vi "AutoCAD NET cmds.vi"(6 "AutoCAD cmd":T3, 8 "error in (no error)":errorcluster, 9 "progress":refnum<vi>, 10 "Mathcad Output":T2, 11 "DesignRequest":T1) -> (0 "error out":errorcluster, 3 "DesignRequest out":T1)   [LabVIEW 2012, in "Design Server.lvlib"]
uses:
  Design Server.lvlib
  AutoCAD cmds.ctl
  Design Request.ctl
  Variable cluster.ctl
  C:/Program Files/Autodesk/AutoCAD 2013/Autodesk.AutoCAD.Interop.dll
  Program Files/Autodesk/AutoCAD 2013/Autodesk.AutoCAD.Interop.dll
panel:
  out "error out 3":errorcluster
  out "error out 2":errorcluster
  out "error array":errorcluster[](array[cluster])
  out "Version":string
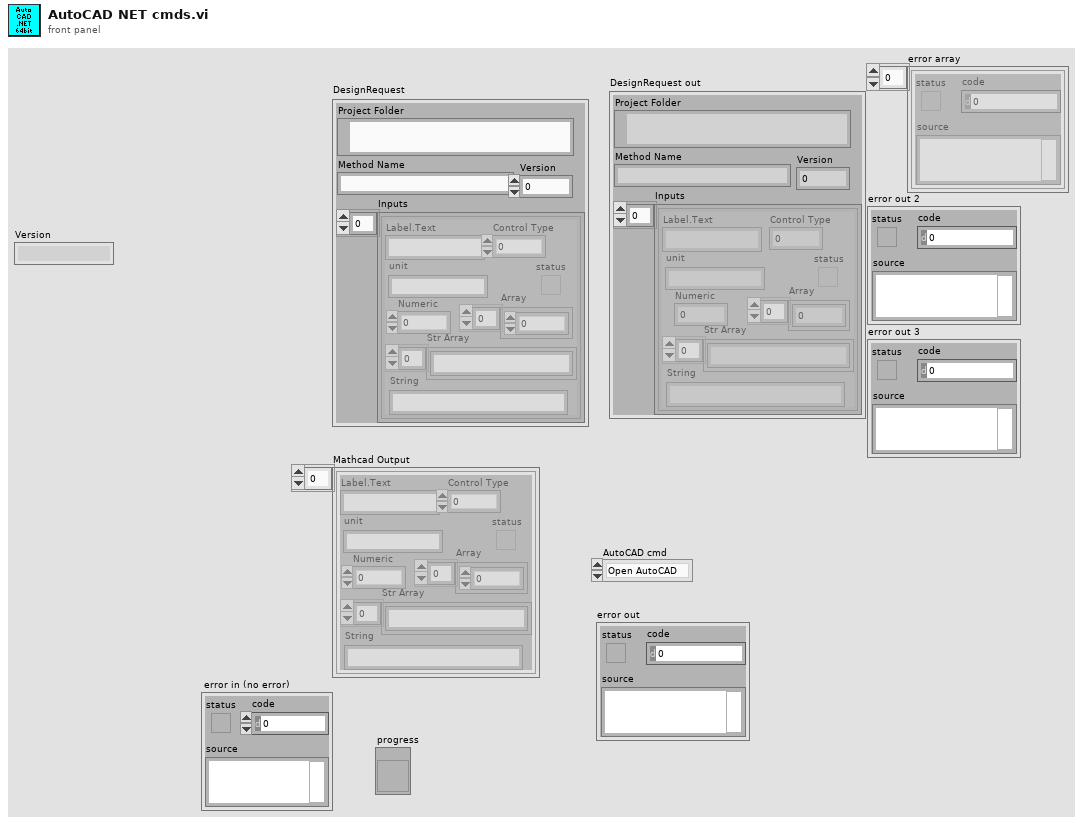
[diagram p1: front panel]
types:
  T1 = typedef "Design Server.lvlib/Design Request.ctl" = cluster{"Project Folder":path, "Method Name":string, "Inputs":T2, "Version":i32}
  T2 = typedef "Design Server.lvlib/Variable cluster.ctl" = cluster{"Label.Text":string, "Control Type":u32, "Numeric":dbl, "Array":dbl[], "status":bool, "Str Array":string[], "String":string, "unit":string}[]
  T3 = typedef "Design Server.lvlib/AutoCAD cmds.ctl" = enum16{"Open AutoCAD", "Create Drawing", "Quit"}
  T4 = typedef "Method.ctl" = cluster{"Title":string, "About":string, "Input Parameters":cluster{"Description":string, "Name":string, "Min":string, "Max":string, "Default":string, "Units":string, "Increment":string, "Stock designs":string[]}[], "AutoCAD drawings":cluster{"File Name":string, "AC Variables":string[]}[], "Stock file names":string[], "Publish files":string[], "Display images":string[]}
  T5 = cluster{"File Name":string, "AC Variables":string[]}[]
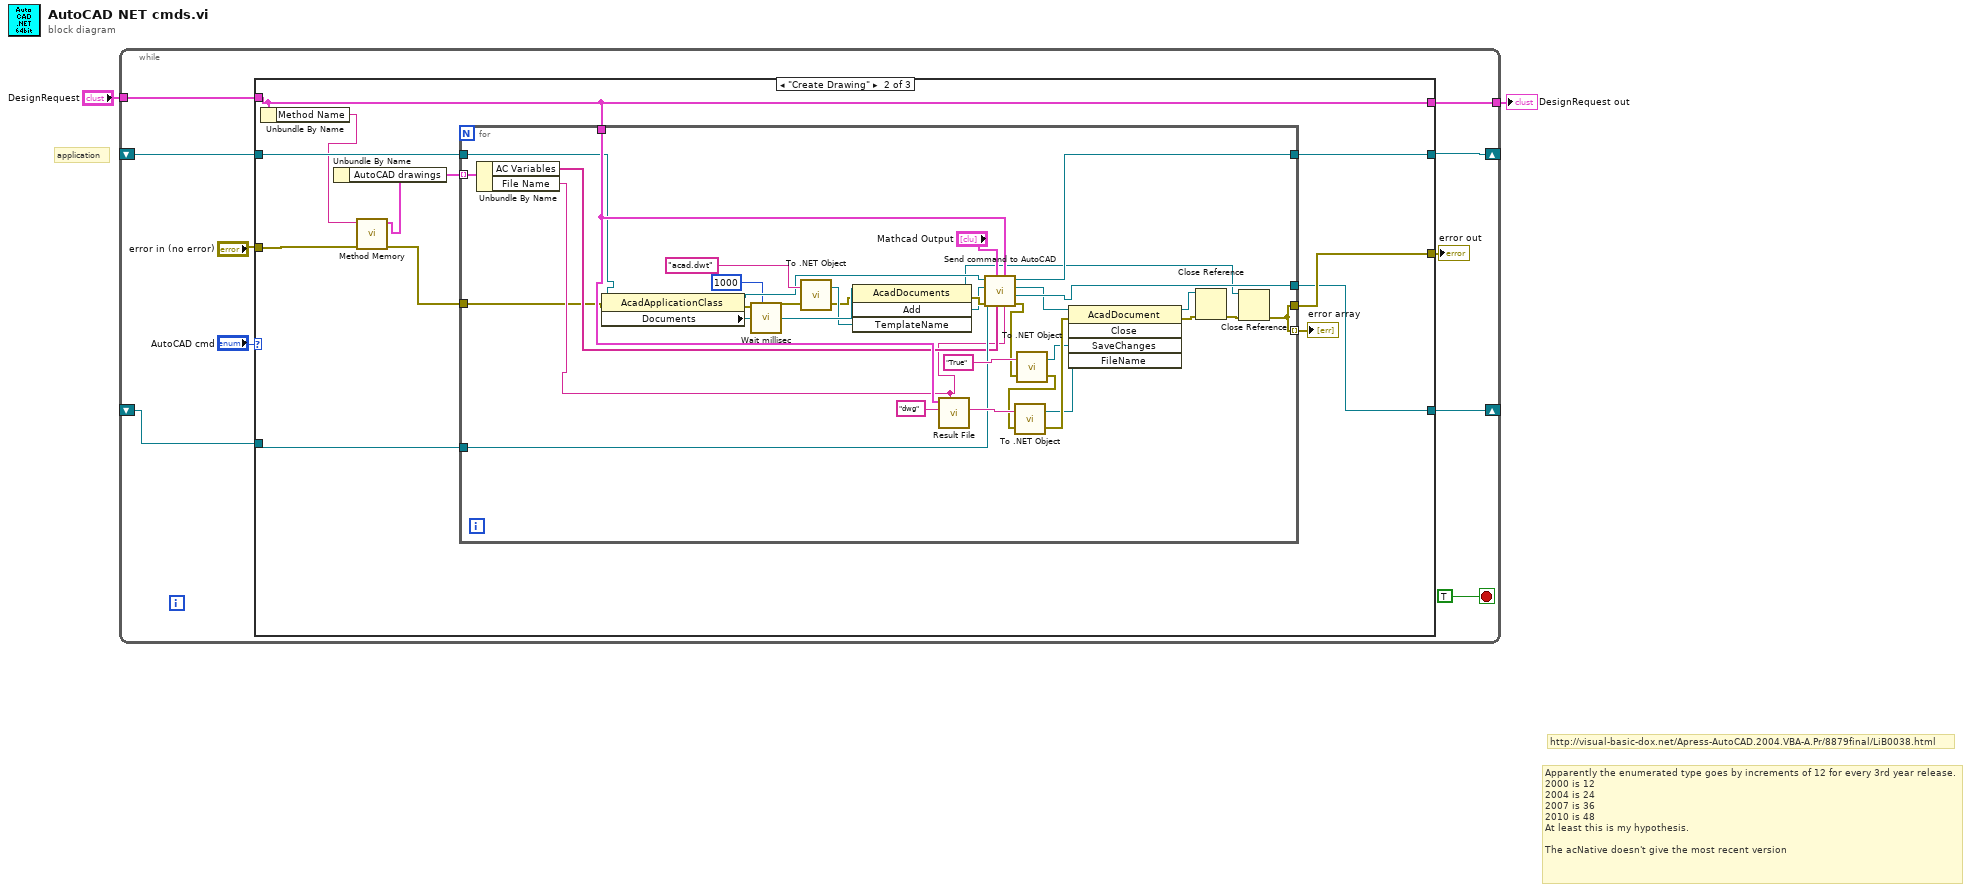
[diagram p0: block diagram]
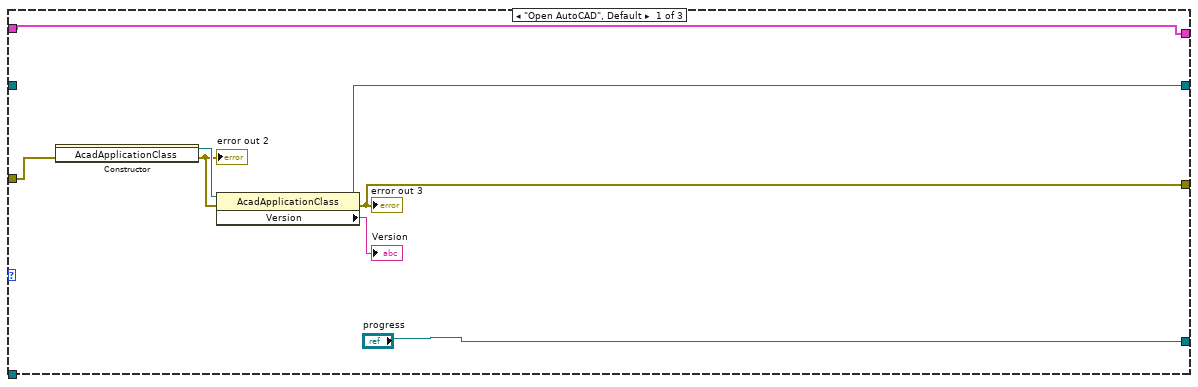
[diagram p2: hidden frame]
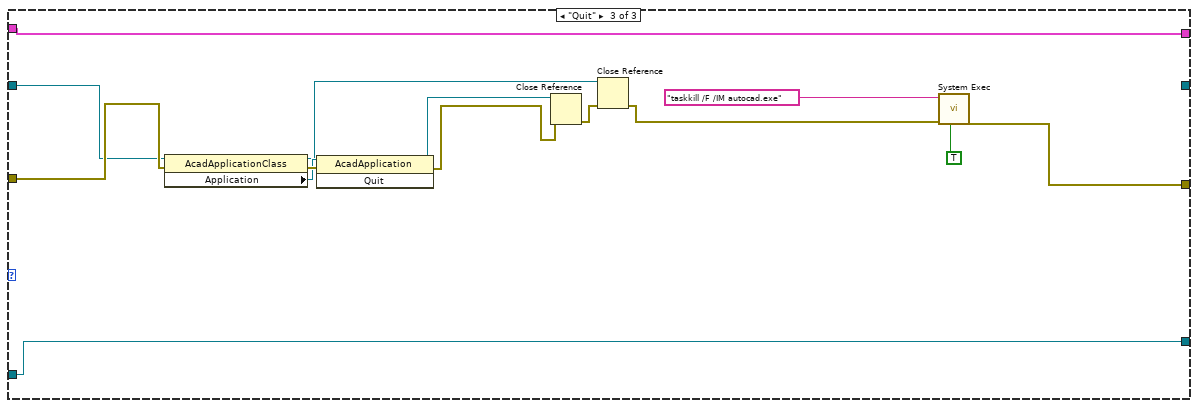
[diagram p3: hidden frame]
diagram:
  # "Apparently the enumerated type goes by increments of 12 for every 3rd year release.\n2000 is 12\n2004 is 24\n2007 is 36\n2010 is 48\nAt least this is my hypothesis. \n\nThe acNative doesn't give the most recent version"
  # "http://visual-basic-dox.net/Apress-AutoCAD.2004.VBA-A.Pr/8879final/LiB0038.html"
  # "application"
  n1 = while {
    shift-right: [w11] -> _
    shift-left: _ -> [w8]
    tunnel: [w6] -> w2
    tunnel: "DesignRequest" -> [w5]
    shift-right: [w4] -> _
    shift-left: _ -> [w3]
    stop <- TRUE stop-if-true
    n2 = case shown="\"Create Drawing\"" "AutoCAD cmd" {
      tunnel: [w17 w27 _] -> w11
      tunnel: "error in (no error)" -> [w13 w22 w75]
      tunnel: [w16 w31 w78] -> w9
      tunnel: w8 -> [_ w32 w72]
      tunnel: [w20 w28 w80] -> w6
      tunnel: w5 -> [w20 w28 w80]
      tunnel: ["progress" w29 w77] -> w4
      tunnel: w3 -> [_ w30 w77]
      frame "Open AutoCAD", Default {
        n3 = constructor class="AcadApplicationClass"(error in=w13) -> (reference out=w15:refnum<k24>, error out=w14:errorcluster)  [unwired: 2 in, 1 out]
        "error out 2" <- w14
        n4 = property class="AcadApplicationClass"(reference=w15, error in=w14) -> (reference out=w17:refnum<k24>, error out=w16:errorcluster, "Version"=→"Version":string)
        "error out 3" <- w16
      }
      frame "Create Drawing" {
        n5 = Unbundle By Name(w28) -> ("Method Name"=w21:string)
        n6 = call "Method Memory.vi"("error in"=w22, "Method Name"=w21) -> ("error out"=w23:errorcluster, "Method Out"=w26:T4)  [unwired: 7 in, 1 out]
        n7 = Unbundle By Name(w26) -> ("AutoCAD drawings"=w25:T5)
        n8 = for {
          tunnel: w23 -> [w52]
          tunnel: w32 -> [w53]
          tunnel: [w37] -> w31
          tunnel: w30 -> [w61]
          tunnel: [w40] -> w29
          tunnel: w28 -> [w60]
          tunnel: [w59] -> w27
          tunnel: w25 -> [w58] mode=indexing
          tunnel: [w37] -> w24 mode=indexing
          n9 = Unbundle By Name(w58) -> ("AC Variables"=w57:string[], "File Name"=w56:string)
          n10 = property class="AcadApplicationClass"(reference=w53, error in=w52) -> (reference out=w51:refnum<k24>, error out=w34:errorcluster, "Documents"=w50:refnum<k24>)
          n11 = call "Wait millisec.vi"("milliseconds to wait"=u32 1000, "error in (no error)"=w34) -> ("error out"=w35:errorcluster)  [unwired: 9 in]
          n12 = call <vilib>:"To .NET Object.vi"("error in (no error)"=w35, "anything"="acad.dwt") -> ("error out"=w48:errorcluster, ".NET object"=w49:refnum<k24>)
          n13 = invoke class="AcadDocuments" method="Add"(reference=w50, error in=w48, "TemplateName"=w49) -> (reference out=w36:refnum<k24>, error out=w47:errorcluster, "Add"=w41:refnum<k24>)  [unwired: 1 in, 1 out]
          n14 = call "Result File.vi"("File name suffix"=w56, "File Type"="dwg", "DesignRequest"=w60) -> ("File string"=w64:string)  [unwired: 7 in, 1 out]
          n15 = call "Send command to AutoCAD.vi"("File name suffix"=w56, "DesignRequest"=w60, "AC Variables"=w57, "Mathcad Output"="Mathcad Output", "error in (no error)"=w47, "progress"=w61, "Add"=w41, "AutoCad app in"=w51) -> ("error out"=w54:errorcluster, "progress out"=w40:refnum<vi>, "Add out"=w39:refnum<k24>, "AutoCad app out"=w59:refnum<k24>)
          n16 = call <vilib>:"To .NET Object.vi"("error in (no error)"=w54, "anything"="True") -> ("error out"=w55:errorcluster, ".NET object"=w44:refnum<k24>)
          n17 = call <vilib>:"To .NET Object.vi"("error in (no error)"=w55, "anything"=w64) -> ("error out"=w46:errorcluster, ".NET object"=w45:refnum<k24>)
          n18 = invoke class="AcadDocument" method="Close"(reference=w39, error in=w46, "SaveChanges"=w44, "FileName"=w45) -> (reference out=w43:refnum<k24>, error out=w42:errorcluster)  [unwired: 1 in, 3 out]
          n19 = Close Reference(reference=w43, error in (no error)=w42) -> (error out=w38:errorcluster)
          n20 = Close Reference(reference=w36, error in (no error)=w38) -> (error out=w37:errorcluster)
        }
        "error array" <- w24
      }
      frame "Quit" {
        n21 = property class="AcadApplicationClass"(reference=w72, error in=w75) -> (reference out=w68:refnum<k24>, error out=w74:errorcluster, "Application"=w71:refnum<k24>)
        n22 = invoke class="AcadApplication" method="Quit"(reference=w71, error in=w74) -> (reference out=w70:refnum<k24>, error out=w73:errorcluster)  [unwired: 1 in, 1 out]
        n23 = Close Reference(reference=w70, error in (no error)=w73) -> (error out=w69:errorcluster)
        n24 = Close Reference(reference=w68, error in (no error)=w69) -> (error out=w67:errorcluster)
        n25 = call <vilib>:"System Exec.vi"("run minimized? (F)"=TRUE, "error in (no error)"=w67, "command line"="taskkill /F /IM autocad.exe") -> ("error out"=w78:errorcluster)  [unwired: 5 in, 3 out]
      }
    }
    "error out" <- w9
  }
  "DesignRequest out" <- w2
